vi "Buffer Data.vi"(8 "error in (no error)":errorcluster, 10 "Data":T1, 11 "Group Buffer DBL in":refnum<class "Group Buffer DBL.lvclass">) -> (0 "error out":errorcluster, 3 "Group Buffer DBL out":refnum<class "Group Buffer DBL.lvclass">)   [LabVIEW 2020, in "VolatusHistorian.lvlib" / "Group Buffer DBL.lvclass"]
uses:
  Group Buffer DBL.lvclass
  lv-vecto/Vecto/Subscribed Data.ctl
  Group Buffer DBL.lvclass/Group Buffer DBL.ctl
  Channel Buffer DBL/Channel Buffer DBL.lvclass/Channel Buffer DBL.ctl
  Channel Buffer DBL/Channel Buffer DBL.lvclass
  lv-vecto/Vecto/Vecto.lvlib
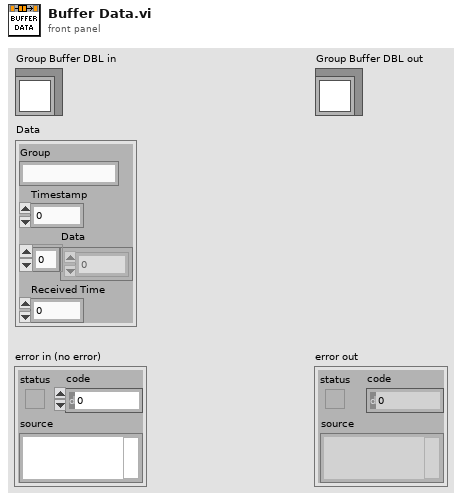
[diagram p1: front panel]
types:
  T1 = typedef "Vecto.lvlib/Subscribed Data.ctl" = cluster{"Group":string, "Timestamp":dbl, "Data":dbl[], "Received Time":dbl}
  T2 = typedef "VolatusHistorian.lvlib/Group Buffer DBL.lvclass/Ref.ctl" = cluster{"Time":refnum<queue>, "Channel Name Map":map{string, i32}, "Group Info":T3, "Channels":refnum<class "Channel Buffer DBL.lvclass">[], "Channel Names":string[]}
  T3 = typedef "VectoConfig.lvlib/Group Info.ctl" = cluster{"System":string, "Cluster":string, "Node":string, "Task":string, "Name":string}
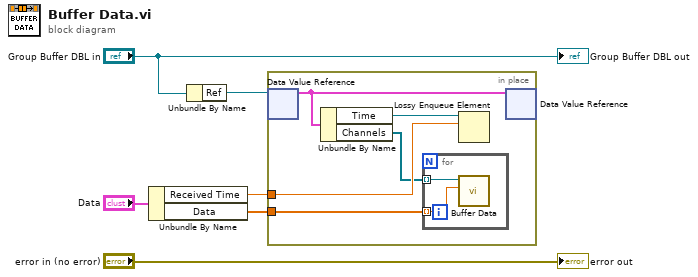
[diagram p0: block diagram]
diagram:
  n1 = Unbundle By Name("Data") -> ("Received Time"=w4:dbl, "Data"=w3:dbl[])
  n2 = Unbundle By Name("Group Buffer DBL in") -> ("Ref"=w1:refnum<data-value>)
  n3 = in-place {
    in-place-border: w4 -> [w10]
    in-place-border: w3 -> [w9]
    n4 = in-place-dvr #1(w1) -> (w7:T2)  [unwired: 1 out]
    n5 = Unbundle By Name(w7) -> ("Time"=w11:refnum<queue>, "Channels"=w8:refnum<class "Channel Buffer DBL.lvclass">[])
    n6 = for {
      tunnel: w8 -> [w13] mode=indexing
      tunnel: w9 -> [w12] mode=indexing
      n7 = call "Buffer Data.vi"("Data"=w12, "Channel Buffer DBL in"=w13) -> ()  [unwired: 8 in, 2 out]
    }
    n8 = Lossy Enqueue Element(queue=w11, element=w10) -> ()  [unwired: 1 in, 4 out]
    n9 = in-place-dvr #1(w7) -> ()  [unwired: 2 out]
  }
  "error out" <- "error in (no error)"
  "Group Buffer DBL out" <- "Group Buffer DBL in"
